vi "MU Get Param.vi"(8 "error in (no error)":errorcluster, 10 "parameter":u32, 11 "MUhandle":u64) -> (0 "error out (no error)":errorcluster, 2 "value":u64, 3 "function return":u32)   [LabVIEW 2017, in "MU_3SL_interface.lvlib"]
uses:
  MU_3SL_interface.lvlib
  lib/MU_3SL_interface.dll
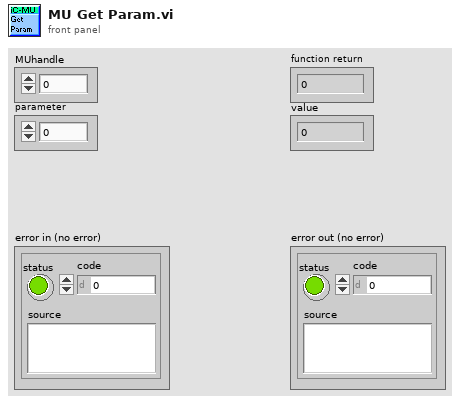
[diagram p1: front panel]
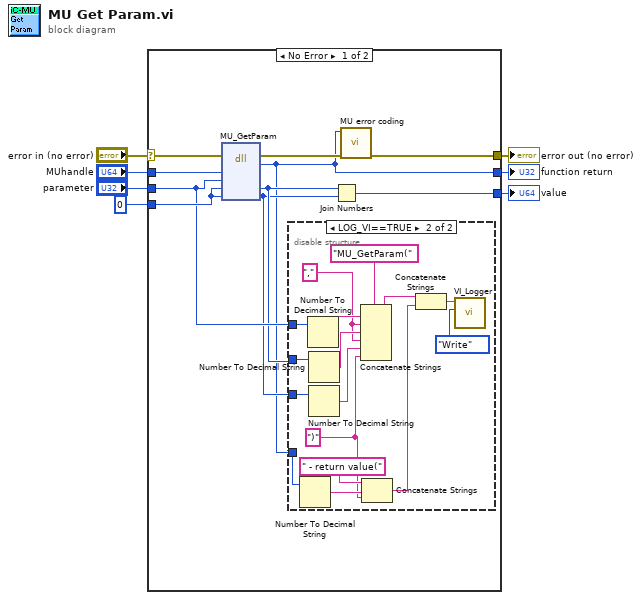
[diagram p0: block diagram]
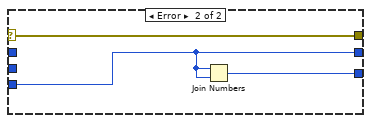
[diagram p3: hidden frame]
diagram:
  n1 = case shown="No Error" "error in (no error)" {
    selector: "error in (no error)" -> [w12 w34]
    tunnel: [w8 w36] -> w7
    tunnel: "MUhandle" -> [w17 _]
    tunnel: "parameter" -> [w11 _]
    tunnel: [w15 w34] -> w4
    tunnel: u32 0 ("pulValueH") -> [w14 w36]
    tunnel: [w13 w35] -> w2
    frame No Error {
      n2 = dll-call lib="C:/Users/sb/AppData/Roaming/work/soft_mu_9so/icsubmodules/soft_mu_3sl_master/lv_interface/lib/MU_3SL_interface**.*" fn="MU_GetParam"(error in=w12, "handle"=w17, "parameter"=w11, "valueHigh"=w14, "valueLow"=w14) -> (error out=w16:errorcluster, "return type"=w8:u32, "valueHigh"=w10:u32, "valueLow"=w9:u32)  [unwired: 4 in, 1 out]
      n3 = disable-structure shown="LOG_VI==TRUE" {
        disable-tunnel: w8 -> [_ w31]
        disable-tunnel: w11 -> [_ w26]
        disable-tunnel: w10 -> [_ w24]
        disable-tunnel: w9 -> [_ w18]
        frame condition #0 {
        }
        frame condition #1 (active) {
          w20 = ")" ("string")
          w21 = "," ("string")
          n4 = Number To Decimal String(number=w31) -> (decimal integer string=w30:string)  [unwired: 1 in]
          n5 = Number To Decimal String(number=w26) -> (decimal integer string=w25:string)  [unwired: 1 in]
          n6 = Number To Decimal String(number=w24) -> (decimal integer string=w23:string)  [unwired: 1 in]
          n7 = Number To Decimal String(number=w18) -> (decimal integer string=w19:string)  [unwired: 1 in]
          n8 = Concatenate Strings("MU_GetParam(" ("Info in"), w25, w21, w23, w21, w19, w20) -> (w29:string)
          n9 = Concatenate Strings(" - return value(" ("string"), w30, w20) -> (w28:string)
          n10 = Concatenate Strings(w29, w28) -> (w27:string)
          n11 = call "VI_Logger.vi"("Action (Read)"=enum16{"Write", "Read"}."Write", "Info in"=w27) -> ()  [unwired: 8 in, 2 out]
        }
      }
      n12 = Join Numbers(hi=w10, lo=w9) -> ((hi.lo)=w13:u64)
      n13 = call "MU error coding.vi"("error in (no error)"=w16, "function return in"=w8) -> ("error out"=w15:errorcluster)  [unwired: 9 in]
    }
    frame Error {
      n14 = Join Numbers(hi=w36, lo=w36) -> ((hi.lo)=w35:u64)
    }
  }
  "function return" <- w7
  "error out (no error)" <- w4
  "value" <- w2
